vi "Data Type Conversion FXP(+-,18,1) to FXP(+-,14,1)x4ch.vi"(4 "data in":T2={[0.0, 0.0], [0.0, 0.0], [0.0, 0.0], [0.0, 0.0]}) -> (0 "overflow":bool, 1 "data out":T1)   [LabVIEW 2015]
doc: "Converts data type from one format to another. The acceptable data types are: +- FXP 18,1; +-, FXP 14,1; and I16.\n\n<B>Supported data types</B>\nFXP +-,18,1; FXP +-,14,1; I16\n\n<B>Supported channel size</B>\n4, 8\n\n<B>Supported samples per cycle</B>\n2\n\n<B>Input Parameters</B>\n\n<B>data in</B> specifies the data to convert to another data type.\n\n<B>Output Parameters</B>\n\n<B>data out</B> returns the converted data.\n\n<B>overflow</B> returns the overflow carried through the data path."
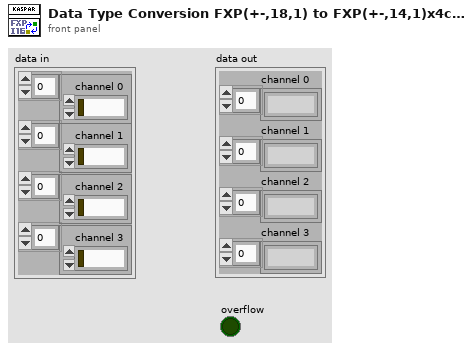
[diagram p1: front panel]
types:
  T1 = cluster{"channel 0":fxp<+/-,14,1>[], "channel 1":fxp<+/-,14,1>[], "channel 2":fxp<+/-,14,1>[], "channel 3":fxp<+/-,14,1>[]}
  T2 = cluster{fxp<+/-,18,1>[], fxp<+/-,18,1>[], fxp<+/-,18,1>[], fxp<+/-,18,1>[]}
  T3 = cluster{"data out":fxp<+/-,14,1>[], "data out":fxp<+/-,14,1>[], "data out":fxp<+/-,14,1>[], "data out":fxp<+/-,14,1>[]}
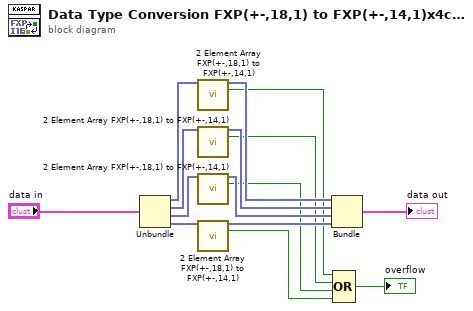
[diagram p0: block diagram]
diagram:
  n1 = Unbundle("data in") -> (w14:fxp<+/-,18,1>[], w12:fxp<+/-,18,1>[], w10:fxp<+/-,18,1>[], w8:fxp<+/-,18,1>[])
  n2 = call "2 Element Array FXP(+-,18,1) to FXP(+-,14,1).vi"("data in"=w14) -> ("data out"=w13:fxp<+/-,14,1>[], "overflow"=w6:bool)  [unwired: 13 in]
  n3 = call "2 Element Array FXP(+-,18,1) to FXP(+-,14,1).vi"("data in"=w12) -> ("data out"=w11:fxp<+/-,14,1>[], "overflow"=w5:bool)  [unwired: 13 in]
  n4 = call "2 Element Array FXP(+-,18,1) to FXP(+-,14,1).vi"("data in"=w10) -> ("data out"=w9:fxp<+/-,14,1>[], "overflow"=w4:bool)  [unwired: 13 in]
  n5 = call "2 Element Array FXP(+-,18,1) to FXP(+-,14,1).vi"("data in"=w8) -> ("data out"=w7:fxp<+/-,14,1>[], "overflow"=w3:bool)  [unwired: 13 in]
  n6 = Bundle("data out"=w13, "data out"=w11, "data out"=w9, "data out"=w7) -> (→"data out":T3)  [unwired: 1 in]
  n7 = Compound Arithmetic op=OR(w6, w5, w4, w3) -> (→"overflow":bool)
